vi "Format Flow vs Current.vi"(0 "Current Step ID":i32, 1 "Flow":dbl, 2 "Current":dbl) -> ()   [LabVIEW 2018]
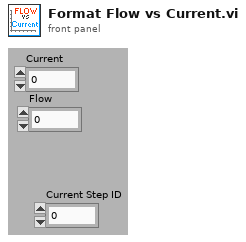
[diagram p1: front panel]
types:
  T1 = enum16{"get data", "set data", "Add Data Pair", "initialize"}
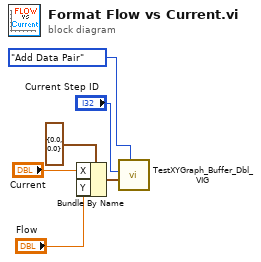
[diagram p0: block diagram]
diagram:
  n1 = Bundle By Name(cluster=cluster{"X":dbl, "Y":dbl} {"X"=0.0, "Y"=0.0} ("XYCluster"), "X"="Current", "Y"="Flow") -> (w6:cluster{"X":dbl, "Y":dbl})
  n2 = call "TestXYGraph_Buffer_Dbl_VIG.vi"("Operation"=T1."Add Data Pair", "XYCluster"=w6, "index/size"="Current Step ID") -> ()  [unwired: 7 in, 2 out]
